vi "Altitude Facade.vi"(0 "Data In":T6, 2 "Display State In":T4, 3 "Container State":T5) -> (6 "Data Out":T6, 7 "Display State Out":T4, 8 "Action":T3)   [LabVIEW 2013, in "Altitude.xctl"]
uses:
  Altitude.xctl
  Altitude Data.ctl
  <vilib>/_xctls/Container State.ctl
  Altitude State.ctl
  <vilib>/_xctls/Action.ctl
  Type Defs/Alt Control small.ctl
  Type Defs/Alt Digit 36 New.ctl
  <vilib>/_xctls/XControlSupport.lvlib
panel:
  in  "Alt Ctl":T1 {"?" min=0 max=9 step=1; "?" min=0 max=9 step=1; "?" min=0 max=9 step=1; "?" min=0 max=9 step=1; "?" min=0 max=9 step=1}
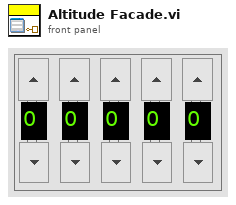
[diagram p1: front panel]
types:
  T1 = typedef "Alt Control small.ctl" = cluster{T2, T2, T2, T2, T2}
  T2 = typedef "Alt Digit 36 New.ctl" = i8
  T3 = typedef "XControlSupport.lvlib/Action.ctl" = cluster{"Data Changed?":bool, "State Changed?":bool, "Action Name":string}
  T4 = typedef "Altitude.xctl/Altitude State.ctl" = cluster{"Numeric":dbl}
  T5 = typedef "XControlSupport.lvlib/Container State.ctl" = cluster{"Indicator?":bool, "Run Mode?":bool, " Refnum":refnum<vi>}
  T6 = typedef "Altitude.xctl/Altitude Data.ctl" = sgl
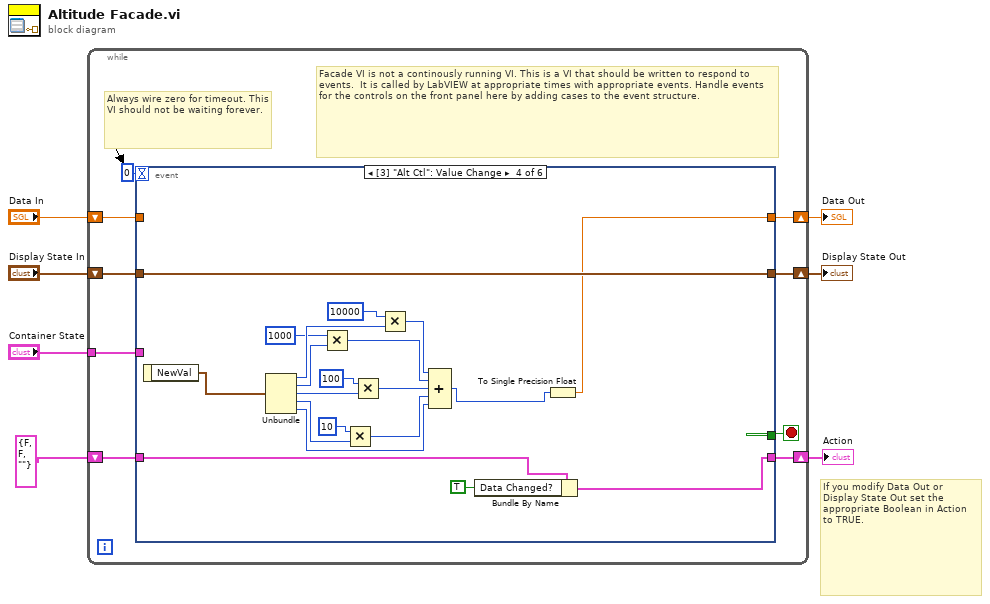
[diagram p0: block diagram]
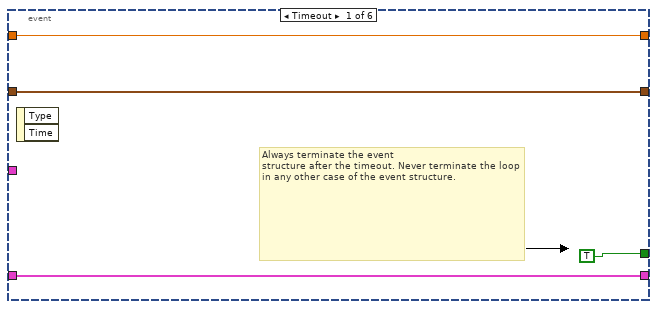
[diagram p2: hidden frame]
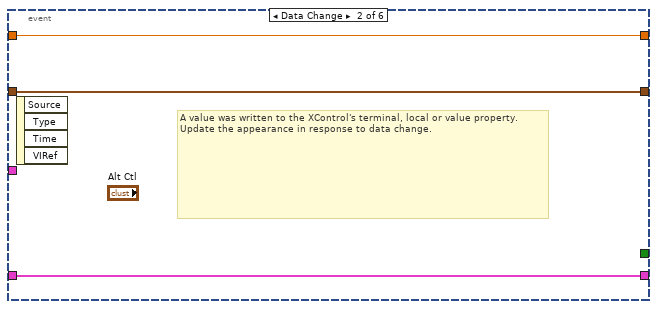
[diagram p3: hidden frame]
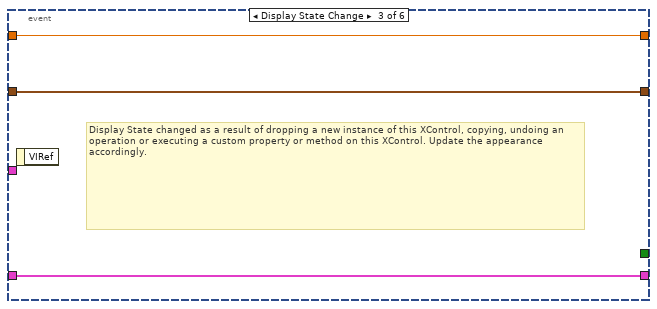
[diagram p4: hidden frame]
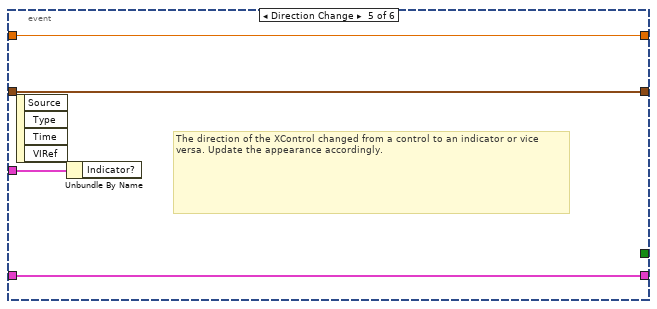
[diagram p5: hidden frame]
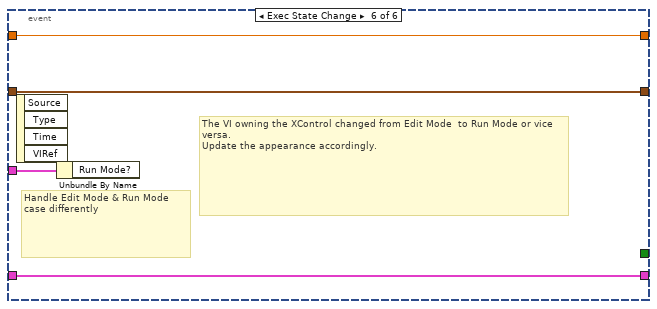
[diagram p6: hidden frame]
diagram:
  # "If you modify Data Out or\nDisplay State Out set the\nappropriate Boolean in Action\nto TRUE."
  n1 = while {
    shift-right: [w15] -> w4
    shift-left: "Display State In" -> [w16]
    tunnel: "Container State" -> [w12]
    shift-right: [w10] -> w7
    shift-left: "Data In" -> [w11]
    shift-right: [w8] -> w2
    shift-left: T3 {"Data Changed?"=FALSE, "State Changed?"=FALSE, "Action Name"=""} ("Action") -> [w9]
    stop <- w14 stop-if-true
    # "Facade VI is not a continously running VI. This is a VI that should be written to respond to events.  It is called by LabVIEW at appropriate times with appropriate events. Handle events for the controls on the front panel here by adding cases to the event structure."
    # "Always wire zero for timeout. This\nVI should not be waiting forever."
    n2 = event shown="[3] \"Alt Ctl\": Value Change" {
      selector: _ -> [_ _ _ _ _ _]
      dyn-events: _ -> [_ _ _ _ _ _]
      timeout: 0 -> [_ _ _ _ _ _]
      tunnel: w16 -> [w18 w22 w26 w46 w49 w53]
      tunnel: [w18 w22 w26 w46 w49 w53] -> w15
      tunnel: [TRUE _ _ _ _ _] -> w14
      tunnel: w12 -> [_ _ _ _ w50 w54]
      tunnel: w11 -> [w17 w23 w25 _ w48 w52]
      tunnel: [w17 w23 w25 w30 w48 w52] -> w10
      tunnel: [w19 w21 w24 w27 w47 w51] -> w8
      tunnel: w9 -> [w19 w21 w24 w29 w47 w51]
      event Timeout {
        # "Always terminate the event\nstructure after the timeout. Never terminate the loop in any other case of the event structure."
        n3 = event-data() -> ()  [unwired: 1 in, 2 out]
      }
      event Data Change {
        # "A value was written to the XControl's terminal, local or value property.\nUpdate the appearance in response to data change."
        n4 = event-data() -> ()  [unwired: 1 in, 4 out]
      }
      event Display State Change {
        # "Display State changed as a result of dropping a new instance of this XControl, copying, undoing an operation or executing a custom property or method on this XControl. Update the appearance accordingly."
        n5 = event-data() -> ()  [unwired: 1 in, 1 out]
      }
      event Value Change {
        n6 = event-data() -> ("NewVal"=w31:T1)  [unwired: 1 in]
        n7 = Unbundle(w31) -> (w45:T2, w40:T2, w39:T2, w38:T2, w33:T2)
        n8 = Multiply(x=u32 1000, y=w40) -> (x*y=w36:u32)
        n9 = Multiply(x=u32 10, y=w38) -> (x*y=w34:u32)
        n10 = Multiply(x=u32 100, y=w39) -> (x*y=w35:u32)
        n11 = Multiply(x=u32 10000, y=w45) -> (x*y=w37:u32)
        n12 = Compound Arithmetic op=ADD(w37, w36, w35, w34, w33) -> (w32:u32)
        n13 = Bundle By Name(cluster=w29, "Data Changed?"=TRUE) -> (w27:T3)
        n14 = To Single Precision Float(number=w32) -> (single precision float=w30:sgl)
      }
      event Direction Change {
        # "The direction of the XControl changed from a control to an indicator or vice versa. Update the appearance accordingly."
        n15 = event-data() -> ()  [unwired: 1 in, 4 out]
        n16 = Unbundle By Name(w50) -> ()  [unwired: 1 out]
      }
      event Exec State Change {
        # "The VI owning the XControl changed from Edit Mode  to Run Mode or vice versa.\nUpdate the appearance accordingly."
        # "Handle Edit Mode & Run Mode\ncase differently"
        n17 = event-data() -> ()  [unwired: 1 in, 4 out]
        n18 = Unbundle By Name(w54) -> ()  [unwired: 1 out]
      }
    }
  }
  "Display State Out" <- w4
  "Data Out" <- w7
  "Action" <- w2
